vi "Get line states.vi"(8 "error in (no error)":errorcluster, 11 "TTL in":refnum<class "TTL.lvclass">) -> (0 "error out":errorcluster, 2 "Current line states":bool[](array[boolean]), 3 "TTL out":refnum<class "TTL.lvclass">)   [LabVIEW 2011, in "TTL.lvclass"]
uses:
  TTL.lvclass
  TTL.lvclass/TTL.ctl
  <vilib>/DAQmx/read.llb/DAQmx Read (Digital 1D Bool NChan 1Samp 1Line).vi
  <vilib>/DAQmx/miscellaneous.llb/DAQmx Fill In Error Info.vi
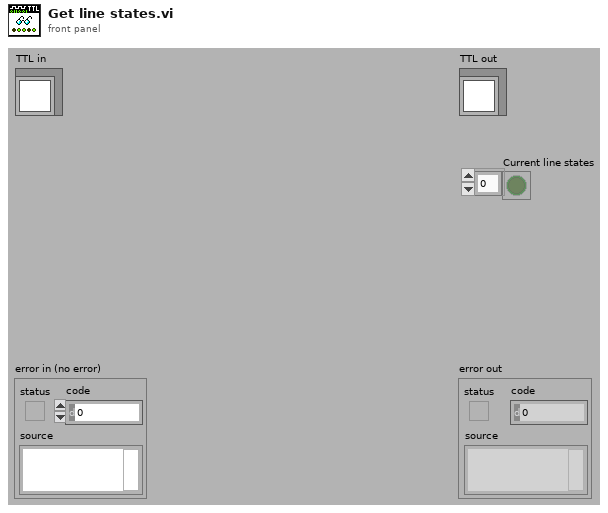
[diagram p1: front panel]
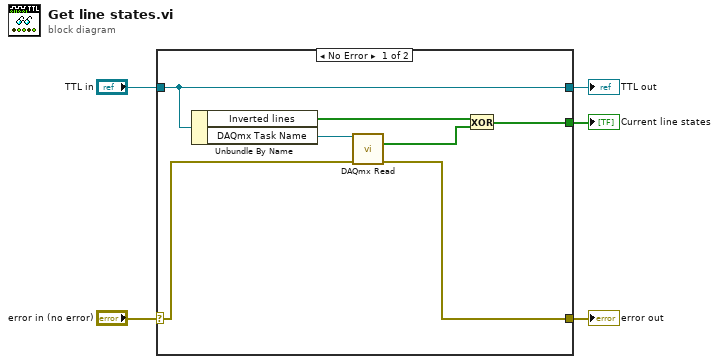
[diagram p0: block diagram]
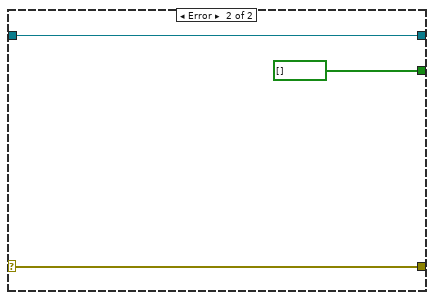
[diagram p2: hidden frame]
diagram:
  n1 = case shown="No Error" "error in (no error)" {
    selector: "error in (no error)" -> [w11 w15]
    tunnel: [w10 w15] -> w4
    tunnel: [w12 w14] -> w2
    tunnel: "TTL in" -> [w12 w14]
    tunnel: [w6 bool[] [] ("data")] -> w1
    frame No Error {
      n2 = Unbundle By Name(w12) -> ("Inverted lines"=w7:bool[], "DAQmx Task Name"=w9:refnum<k21>)
      n3 = call-poly <vilib>:"DAQmx Read.vi"("task/channels in"=w9, "error in"=w11) -> ("data"=w8:bool[], "error out"=w10:errorcluster)  [unwired: 11 in, 1 out]
      n4 = Exclusive Or(1:w8, 2:w7) -> (0:w6:bool[])
    }
    frame Error {
    }
  }
  "error out" <- w4
  "TTL out" <- w2
  "Current line states" <- w1
